vi "Reset.vi"(8 "error in (no error)":errorcluster, 11 "Map in":refnum<class "Map.lvclass">) -> (0 "error out":errorcluster, 3 "Map out":refnum<class "Map.lvclass">)   [LabVIEW 2020, in "SquareBattle.lvlib" / "Map.lvclass"]
uses:
  Map.lvclass
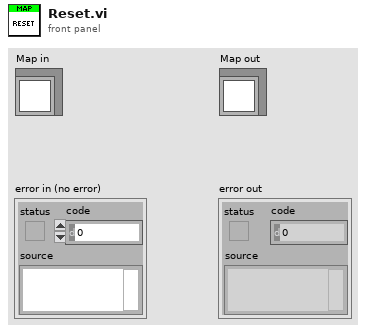
[diagram p1: front panel]
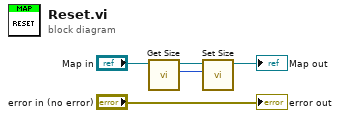
[diagram p0: block diagram]
diagram:
  n1 = call "Get Size.vi"("Map in"="Map in") -> ("Size"=w2:i32, "Map out"=w3:refnum<class "Map.lvclass">)  [unwired: 9 in]
  n2 = call "Set Size.vi"("Size"=w2, "Map in"=w3) -> ("Map out"=→"Map out":refnum<class "Map.lvclass">)  [unwired: 8 in, 1 out]
  "error out" <- "error in (no error)"
